vi "clone.vi"(0 "reference":refnum<class "UseCaseNode.lvclass">, 5 "error in (no error)":errorcluster) -> (14 "reference out":refnum<class "UseCaseNode.lvclass">, 15 "clonedInterfaceNode":refnum<class "AbstractNode.lvclass">, 19 "error out":errorcluster)   [LabVIEW 2016, in "UseCaseNode.lvclass"]
doc: "public Object clone()"
uses:
  <resource>/Framework/Providers/Open_GDS/UML/UseCaseNode_class/UseCaseNode.lvclass
  C:/Program Files (x86)/National Instruments/LabVIEW 2016/resource/Framework/Providers/Open_GDS/UML/RectangularNode_class/RectangularNode.lvclass
  C:/Program Files (x86)/National Instruments/LabVIEW 2016/resource/Framework/Providers/Open_GDS/UML/AbstractNode_class/AbstractNode.lvclass
  <resource>/Framework/Providers/Open_GDS/UML/AbstractNode_class/AbstractNode.lvclass
  <resource>/Framework/Providers/Open_GDS/UML/MultiLineString_class/MultiLineString.lvclass
  <resource>/Framework/Providers/Open_GDS/UML/RectangularNode_class/RectangularNode.lvclass
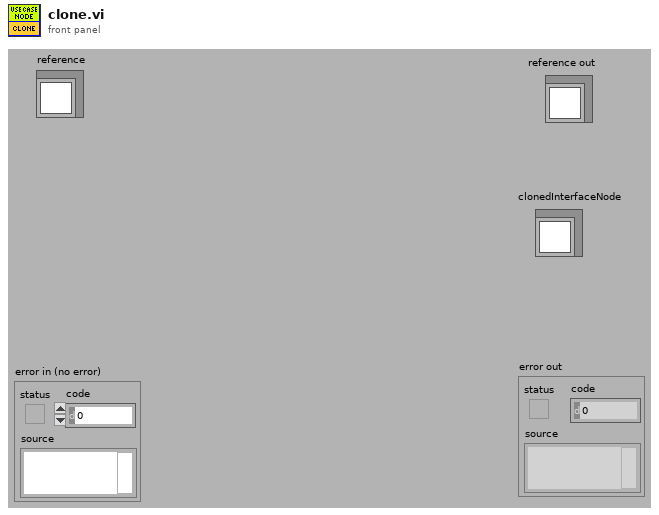
[diagram p1: front panel]
types:
  T1 = typedef "RectangularNode.lvclass/ObjectAttributes.ctl" = cluster{"bounds":T2}
  T2 = typedef "Rectangle Rectangle2D.ctl" = cluster{"x":dbl, "y":dbl, "width":dbl, "height":dbl}
  T3 = typedef "UseCaseNode.lvclass/ObjectAttributes.ctl" = cluster{"name":refnum<class "MultiLineString.lvclass">, "DEFAULT_WIDTH":i32, "DEFAULT_HEIGHT":i32}
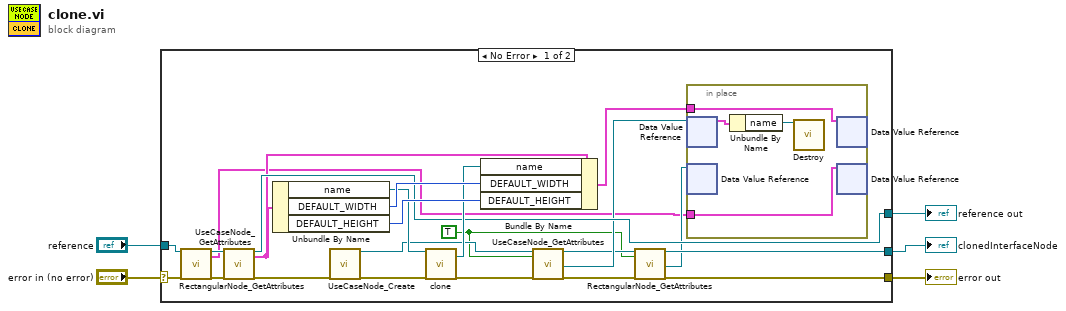
[diagram p0: block diagram]
diagram:
  n1 = case shown="No Error" "error in (no error)" {
    selector: "error in (no error)" -> [w28 w33]
    tunnel: "reference" -> [w13 w34]
    tunnel: [w11 w33] -> w4
    tunnel: [w20 w34] -> w3
    tunnel: [w9 _] -> w1
    frame No Error {
      w6 = TRUE ("OnlyGetDvrReference(False)")
      n2 = call <resource>:"RectangularNode_GetAttributes.vi"("reference in"=w13, "error in (no error)"=w28) -> ("reference out"=w12:refnum<class "UseCaseNode.lvclass">, "Data"=w7:T1, "error out"=w14:errorcluster)  [unwired: 14 in, 1 out]
      n3 = call <resource>:"UseCaseNode_GetAttributes.vi"("reference in"=w12, "error in (no error)"=w14) -> ("reference out"=w20:refnum<class "UseCaseNode.lvclass">, "Data"=w18:T3, "error out"=w19:errorcluster)  [unwired: 1 in, 14 out]
      n4 = Unbundle By Name(w18) -> ("name"=w24:refnum<class "MultiLineString.lvclass">, "DEFAULT_WIDTH"=w27:i32, "DEFAULT_HEIGHT"=w26:i32)
      n5 = call <resource>:"UseCaseNode_Create.vi"("error in (no error)"=w19) -> ("reference out"=w21:refnum<class "UseCaseNode.lvclass">, "error out"=w25:errorcluster)  [unwired: 17 in]
      n6 = call-dynamic "clone.vi"("reference"=w24, "error in (no error)"=w25) -> ("clonedMultiLineString"=w23:refnum<class "MultiLineString.lvclass">, "error out"=w22:errorcluster)  [unwired: 15 in, 1 out]
      n7 = Bundle By Name(cluster=w18, "name"=w23, "DEFAULT_WIDTH"=w27, "DEFAULT_HEIGHT"=w26) -> (w15:T3)
      n8 = call <resource>:"UseCaseNode_GetAttributes.vi"("reference in"=w21, "OnlyGetDvrReference(False)"=w6, "error in (no error)"=w22) -> ("reference out"=w10:refnum<class "UseCaseNode.lvclass">, "DataRef"=w16:refnum<data-value>, "error out"=w17:errorcluster)  [unwired: 13 in, 1 out]
      n9 = call <resource>:"RectangularNode_GetAttributes.vi"("reference in"=w10, "OnlyGetDvrReference(False)"=w6, "error in (no error)"=w17) -> ("reference out"=w9:refnum<class "UseCaseNode.lvclass">, "DataRef"=w8:refnum<data-value>, "error out"=w11:errorcluster)  [unwired: 13 in, 1 out]
      n10 = in-place {
        in-place-border: w15 -> [w32]
        in-place-border: w7 -> [w29]
        n11 = in-place-dvr #1(w16) -> (w30:T3)  [unwired: 1 out]
        n12 = in-place-dvr #2(w8) -> ()  [unwired: 2 out]
        n13 = Unbundle By Name(w30) -> ("name"=w31:refnum<class "MultiLineString.lvclass">)
        n14 = call-dynamic "Destroy.vi"("reference"=w31) -> ()  [unwired: 17 in, 2 out]
        n15 = in-place-dvr #1(w32) -> ()  [unwired: 2 out]
        n16 = in-place-dvr #2(w29) -> ()  [unwired: 2 out]
      }
    }
    frame Error {
    }
  }
  "reference out" <- w3
  "error out" <- w4
  "clonedInterfaceNode" <- w1
